vi "sense_amplitudes.vi"(11 "Ref carrier amplitudes in":T1 format="%#_3p") -> (3 "Sense amplitudes":cdb[][](array[numeric]))   [LabVIEW 2014]
uses:
  carrier_amplitudes.ctl
panel:
  # "High/low"
  # "Source XYZ"
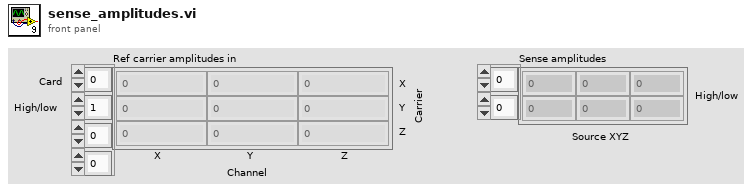
[diagram p1: front panel]
types:
  T1 = typedef "carrier_amplitudes.ctl" = cdb[][][][]
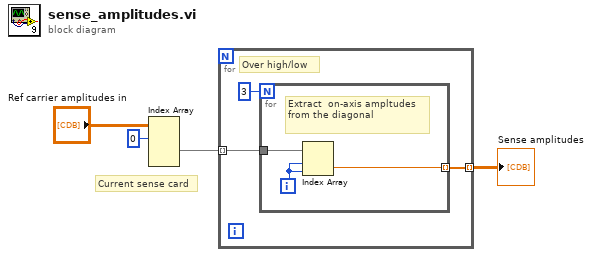
[diagram p0: block diagram]
diagram:
  # "Current sense card"
  n1 = Index Array(array="Ref carrier amplitudes in", index (dim 0)=0 ("index (page)")) -> (element=w2:cdb[][][])  [unwired: 3 in]
  n2 = for {
    tunnel: w2 -> [w7] mode=indexing
    tunnel: [w6] -> w1 mode=indexing
    # "Over high/low"
    n3 = for {
      N: 3 -> [_]
      tunnel: w7 -> [w10]
      tunnel: [w8] -> w6 mode=indexing
      i -> [w9]
      # "Extract  on-axis ampltudes from the diagonal"
      n4 = Index Array(array=w10, index (row)=w9, index (col)=w9) -> (element=w8:cdb)
    }
  }
  "Sense amplitudes" <- w1
